vi "comand_counter.vi"(0 "R":bool, 1 "такты":bool, 2 "Set":T1) -> (3 "q4":bool, 4 "q3":bool, 5 "q2":bool, 6 "q1":bool)   [LabVIEW 2013]
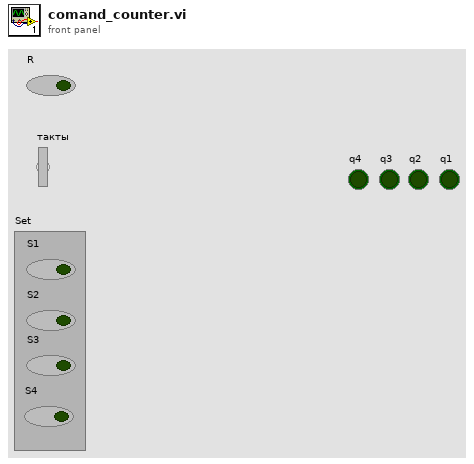
[diagram p1: front panel]
types:
  T1 = cluster{"S1":bool, "S2":bool, "S3":bool, "S4":bool}
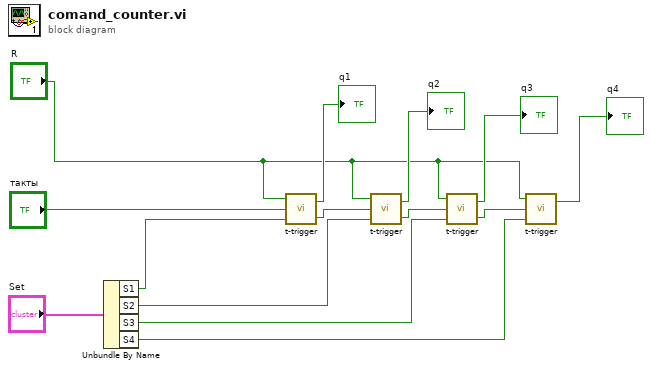
[diagram p0: block diagram]
diagram:
  n1 = Unbundle By Name("Set") -> ("S1"=w4:bool, "S2"=w3:bool, "S3"=w2:bool, "S4"=w1:bool)
  n2 = call "t-trigger.vi"("S"=w4, "T"="такты", "R"="R") -> ("notQ"=w13:bool, "Q"=→"q1":bool)
  n3 = call "t-trigger.vi"("S"=w3, "T"=w13, "R"="R") -> ("notQ"=w12:bool, "Q"=→"q2":bool)
  n4 = call "t-trigger.vi"("S"=w2, "T"=w12, "R"="R") -> ("notQ"=w11:bool, "Q"=→"q3":bool)
  n5 = call "t-trigger.vi"("S"=w1, "T"=w11, "R"="R") -> ("Q"=→"q4":bool)  [unwired: 1 out]
